vi "Initialize.vi"   [LabVIEW 2016, in "SLSC Switch.lvlib" / "SLSC Switch.lvclass"]
uses:
  SLSC Switch.lvclass
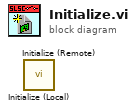
[diagram p0: block diagram]
diagram:
  n1 = call "Initialize (Local).vi"() -> ()  [unwired: 14 in, 2 out]
  n2 = call "Initialize (Remote).vi"() -> ()  [unwired: 14 in, 2 out]
